vi "CheckVoltageImproperWiring.vi"(9 "Wiring Configuration":string, 10 "nominal voltage":dbl, 11 "Group Phasors":T1[](array[typedef])) -> (1 "valid?":bool, 3 "wiring information":string)   [LabVIEW 2017, in "McsaAnalysisLowRate.lvlib"]
uses:
  <vilib>/addons/InsightCM/Devices/Shared/Mcsa/McsaAnalysisLowRate/McsaAnalysisLowRate.lvlib
  <vilib>/addons/InsightCM/Utilities/Analysis/MCSA/controls/McsaChannelPhasor.ctl
  <vilib>/addons/Electrical Power/Basic/NI_EP_Basic.lvlib
  <vilib>/addons/InsightCM/Utilities/Analysis/MCSA/McsaAnalysisFunctions.lvlib
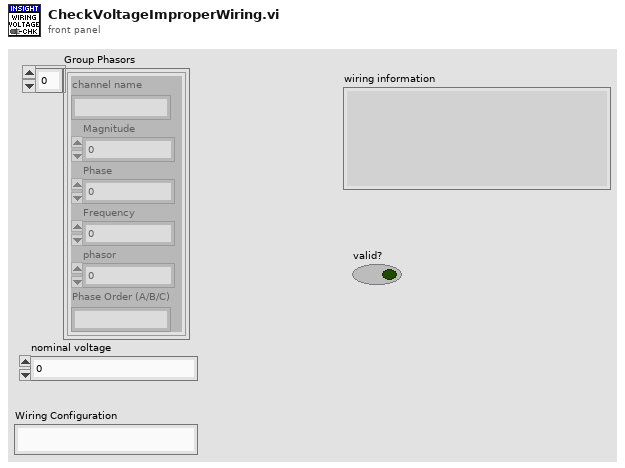
[diagram p1: front panel]
types:
  T1 = typedef "McsaAnalysisFunctions.lvlib/McsaChannelPhasor.ctl" = cluster{"channel name":string, "Magnitude":dbl, "Phase":dbl, "Frequency":dbl, "phasor":cdb, "Phase Order (A/B/C)":string}
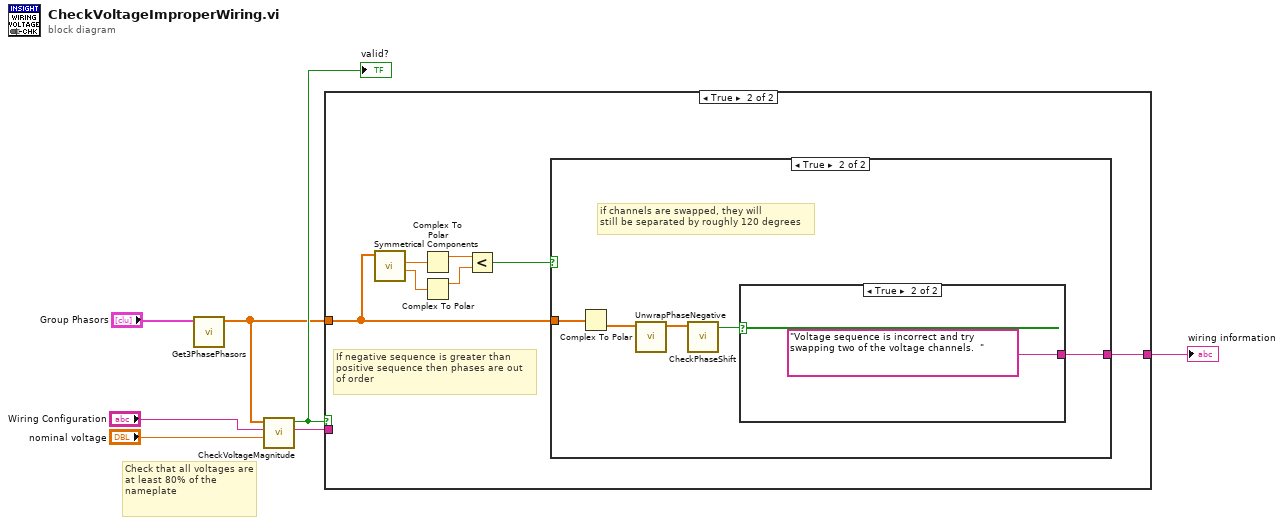
[diagram p0: block diagram]
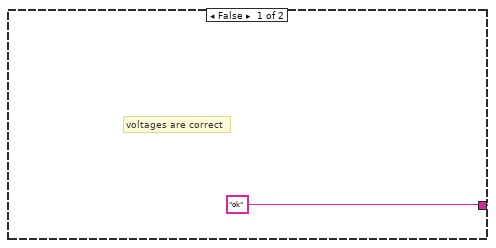
[diagram p3: hidden frame]
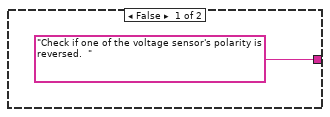
[diagram p4: hidden frame]
diagram:
  # "Check that all voltages are at least 80% of the nameplate"
  n1 = call <vilib>:"Get3PhasePhasors.vi"("Group Phasors"="Group Phasors") -> ("3-phase Phasors"=w2:cdb[])  [unwired: 10 in]
  n2 = call <vilib>:"CheckVoltageMagnitude.vi"("nominal line voltage"="nominal voltage", "Wiring Configuration"="Wiring Configuration", "voltage phasors"=w2) -> ("wiring info"=w1:string, "valid?"=w6:bool)  [unwired: 7 in]
  "valid?" <- w6
  n3 = case shown="True" w6 {
    tunnel: [w8 w10] -> w7
    tunnel: w2 -> [_ w9]
    tunnel: w1 -> [w8 _]
    frame False {
    }
    frame True {
      # "If negative sequence is greater than positive sequence then phases are out of order"
      n4 = call <vilib>:"Symmetrical Components.vi"("3-phase phasors"=w9) -> ("negative sequence"=w12:cdb, "positive sequence"=w13:cdb)  [unwired: 7 in, 2 out]
      n5 = Complex To Polar(r * e^(i*theta)=w13) -> (r=w14:dbl)  [unwired: 1 out]
      n6 = Complex To Polar(r * e^(i*theta)=w12) -> (r=w15:dbl)  [unwired: 1 out]
      n7 = Less?(x=w14, y=w15) -> (x < y?=w11:bool)
      n8 = case shown="True" w11 {
        tunnel: ["ok" w21] -> w10
        tunnel: w9 -> [_ w20]
        frame False {
          # "voltages are correct"
        }
        frame True {
          # "if channels are swapped, they will\nstill be separated by roughly 120 degrees"
          n9 = Complex To Polar(r * e^(i*theta)=w20) -> (theta=w19:dbl[])  [unwired: 1 out]
          n10 = call <vilib>:"UnwrapPhaseNegative.vi"("radian"=w19) -> ("degrees"=w18:dbl[])  [unwired: 10 in]
          n11 = call <vilib>:"CheckPhaseShift.vi"("3-phase phase degree"=w18) -> ("all 120-degree shift?"=w17:bool)  [unwired: 10 in]
          n12 = case shown="True" w17 {
            tunnel: ["Check if one of the voltage sensor's polarity is reversed.  " "Voltage sequence is incorrect and try swapping two of the voltage channels.  "] -> w21
            frame False {
            }
            frame True {
            }
          }
        }
      }
    }
  }
  "wiring information" <- w7
